vi "main.vi"() -> ()   [LabVIEW 2016]
uses:
  Controls/Auto range.ctl
panel:
  out "Waveform Graph":dbl[](graph)
  in  "Phase":dbl format=" %.5f V"
  in  "R":dbl format=" %.5f V"
  in  "Boolean":T1=TRUE
  in  "Range 3":dbl=1.0 caption="Amp" format="%.2p Vpk"
  in  "Range 2":dbl caption="Offest" format="%.2p V"
  in  "Range":dbl(ring)=1.0 items=["10 mV"=0.01, "100 mV"=0.1, "1 V"=1.0, "10 V"=10.0]
  out "Enable":bool
  in  "Rate":dbl=1000.0 format="%#.3p"
  out "Enable":bool
  out "Title_SIG OUT":string
  out "Title_Demodulators":string
  out "Top_Left":bool
  in  "Frequency":dbl=1000000.0 format="%.8p"
  in  "TC":dbl(slide)=0.036603073166094145 scale=0.01..2.0
  in  "Harmonic":dbl=1.0 min=1.0 max=1000.0 step=1.0 format="%#_1g"
  in  "Order":dbl(ring)=4.0 items=["1"=1.0, "2"=2.0, "3"=3.0, "4"=4.0, "5"=5.0, "6"=6.0, "7"=7.0, "8"=8.0]
  out "Title_SIG IN":string
  in  "Range":dbl=1.0 format="%.1p V"
  in  "Reference":u16(ring) items=["Internal Ref", "External Ref/Aux", "External Ref/DIO", "External Ref/Trigger"]
  in  "Reference Source":u16(ring) caption="参考时钟" items=["内部参考时钟", "外部参考时钟/Aux", "外部参考时钟/DIO", "外部参考时钟/Trigger"]
  in  "Offset":dbl format="%#_3p"
  out "Enable":bool
  out "Diff":bool
  out "50 Ω":bool
  out "AC":bool
  # "Data Transfer"
  # "For development only"
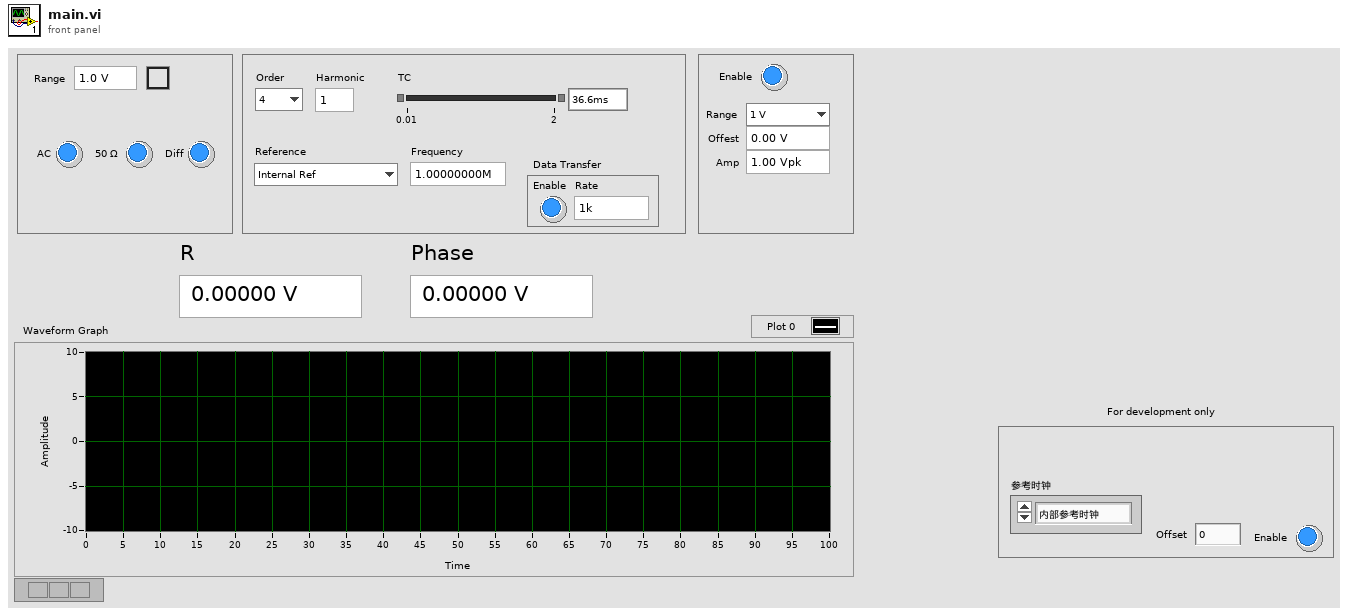
[diagram p1: front panel]
types:
  T1 = typedef "Auto range.ctl" = bool
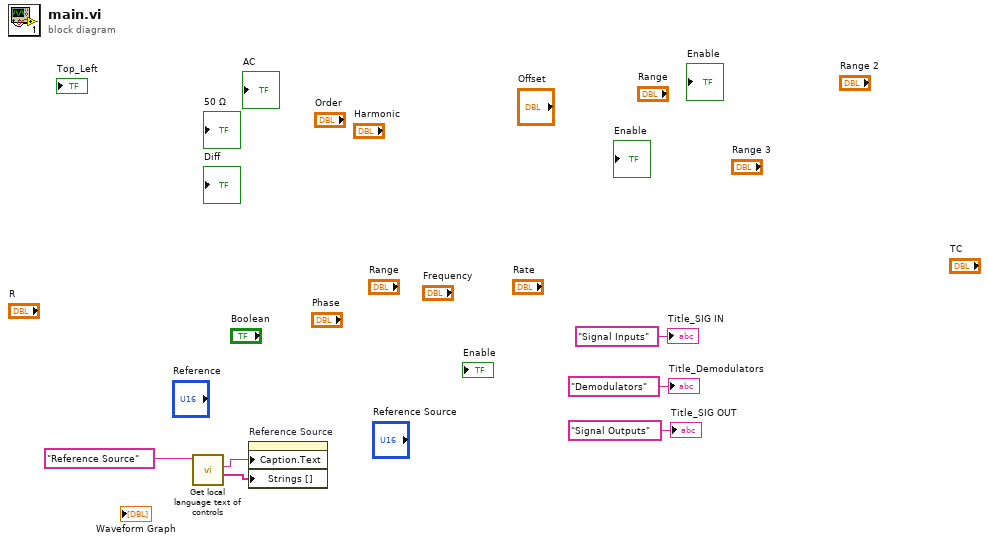
[diagram p0: block diagram]
diagram:
  n1 = call "Get local language text of controls.vi"("Control Label"="Reference Source") -> ("Values"=w5:string[], "Control Caption"=w6:string)  [unwired: 7 in, 2 out]
  n2 = property on="Reference Source" class="Ring (strict)"("Caption.Text"=w6, "Strings []"=w5) -> ()  [unwired: 2 in, 2 out]
  "Title_SIG IN" <- "Signal Inputs" ("Title_SIG IN")
  "Title_Demodulators" <- "Demodulators" ("Title_SIG IN 2")
  "Title_SIG OUT" <- "Signal Outputs" ("Title_SIG OUT")
